vi "Generate LabVIEW FPGA Code for Multistage Multirate Filter.vi"() -> ()   [LabVIEW 2023]
doc: "Demonstrates how to use the DFD FXP NStage MRate Code Generator VI to generate LabVIEW field-programmable gate array (FPGA) code from a fixed-point multistage multirate filter.\n\nComplete the following steps to use this VI.\n1) Specify the <B>Modeling Settings</B>.\n2) Specify a <B>Destination Folder</B> for code generation.\n3) Specify a <B>Filter Name</B> for code generation.\n4) Specify <B># Channels</B> that you want the filter to process.\n5) Specify <B>Open Project?</B> to decide whether to open the generated LabVIEW project or not after code generation.\n6) Run the VI.\n7) Observe the Maximum Input Fs@40 MHz FPGA Clock to obtain information about the processing power of the generated fixed-point multirate filter block."
uses:
  <vilib>/addons/Digital Filter Design/_Objects.llb/DFD Multirate Filtering Mode.ctl
  <vilib>/addons/Digital Filter Design/_Objects.llb/DFD Filter Ripple Specification (Design).ctl
  <vilib>/addons/Digital Filter Design/_Objects.llb/DFD Multirate Filter Specification (Design).ctl
  <vilib>/addons/Digital Filter Design/NI_DigFilterLicensed.lvlib
panel:
  out "Maximum Input Fs@40 MHz FPGA Clock":dbl format="%#_5p Hz"
  out "lvproj Path":path
  in  "Open Project?":bool=TRUE
  in  "Filter Name":string
  in  "# Channels":i32=1
  in  "Destination Folder":path
  out "Error Message":string
  in  "Interstage Word Lengths":i16[](array[numeric])=[16]
  in  "Output Word Length":i16=16
  in  "Input Word Length":i16=16
  # "Select Help>>Show Context Help and move the cursor over the VI icon for more information."
  # "Modeling Settings"
  # "Code Generation Settings"
  # "Code Generation Feedback"
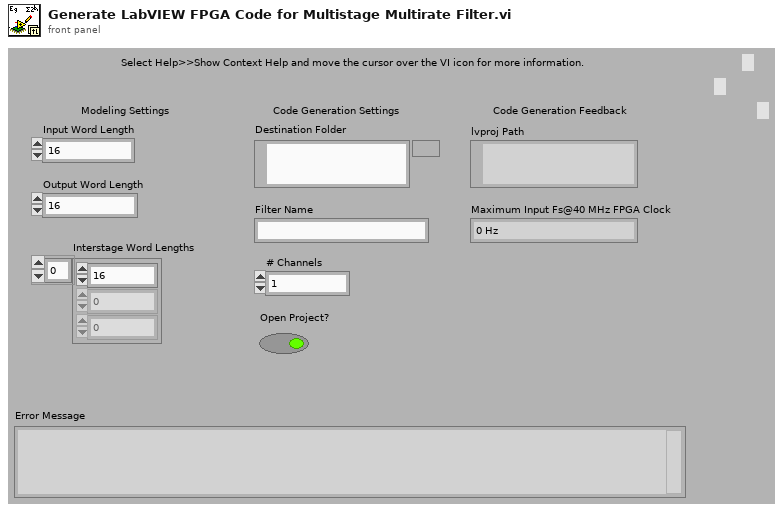
[diagram p1: front panel]
types:
  T1 = typedef "NI_DigFilterLicensed.lvlib/DFD Multirate Filter Specification (Design).ctl" = cluster{"fpass":dbl, "fstop":dbl}
  T2 = typedef "NI_DigFilterLicensed.lvlib/DFD Filter Ripple Specification (Design).ctl" = cluster{"passband":dbl, "stopband":dbl, "dB/linear? (T: dB)":bool}
  T3 = typedef "NI_DigFilterLicensed.lvlib/DFD Multirate Filtering Mode.ctl" = u16
  T4 = typedef "NI_DigFilterLicensed.lvlib/DFD Multirate Filter Obj.ctl" = cluster{"mMRate_Structure":enum16{"CIC", "FIR", "IIR", "Lattice"}, "mMRate_Mode":T5, "mMRate_Factor":i32, "mMRate_FIRParams":cluster{"mMRate_FIR_H":dbl[], "mMRate_FIR_IsNyquist?":bool, "mMRate_FIR_IsSymmetric?":bool}, "mMRate_CICParams":cluster{"mMRate_CIC_#Stage":i32, "mMRate_CIC_Lag":i32, "mMRate_CIC_Type":enum16{"Lowpass", "Highpass"}}, "mMRate_Order":i32, "mMRate_Version":string, "mMRate_Comments":string, "mMRate_RationalFactor":cluster{"mMRate_L":i32, "mMRate_M":i32}, "mMRate_Fs":dbl, "mMRate_Quantized?":bool, "mMRate_QFilterGain":dbl, "mMRate_CoefWl":i16, "mMRate_Scaling":cluster{"mMRate_ScaleByPowerOf2?":bool, "mMRate_ScaleType":T6}, "mMRate_InputWl":i16, "mMRate_OutputWl":i16, "mMRate_OutputMode":T7, "mMRate_MultMode":T8, "mMRate_BitPruning":bool, "mMRate_GainWl":i16, "mMRate_OutputFwl":i16, "mMRate_SumIwl":i16, "mMRate_InputIwl ":i16, "mMRate_SumWl":i16, "mMRate_CoefIwl":i16}
  T5 = typedef "NI_DigFilterLicensed.lvlib/DFD Multirate Mode.ctl" = i16
  T6 = typedef "NI_DigFilterLicensed.lvlib/DFD Coef Norm Type.ctl" = enum16{"No Norm", "Time Domain 1-Norm", "Time Domain 2-Norm", "Time Domain Inf-Norm"}
  T7 = typedef "NI_DigFilterLicensed.lvlib/DFD Round-off Mode.ctl" = enum16{"Nearest", "Truncation"}
  T8 = typedef "NI_DigFilterLicensed.lvlib/DFD FXP MRate Multiply Mode.ctl" = enum16{"Truncated", "Full"}
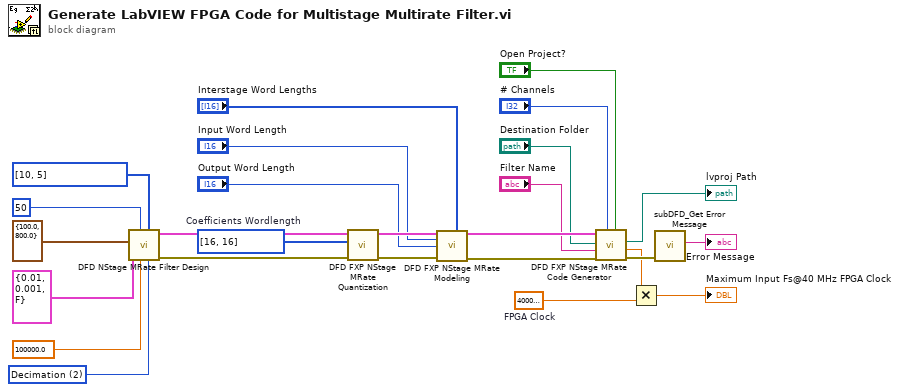
[diagram p0: block diagram]
diagram:
  w4 = 40000000.0  # FPGA Clock
  w18 = i16[] [16, 16]  # Coefficients Wordlength
  w20 = T3 2 items=["No Rate Change", "Interpolation", "Decimation"] ("Filtering Mode")
  n1 = call <vilib>:"DFD NStage MRate Filter Design.vi"("filtering mode"=w20, "manual factorization"=i32[] [10, 5] ("Manual Factorization"), "fs in [Hz]"=100000.0 ("Sampling Rate [Hz]"), "factor"=50 ("Factor"), "ripple specs"=T2 {"passband"=0.01, "stopband"=0.001, "dB/linear? (T: dB)"=FALSE} ("Ripple Specs"), "freq specs [Hz]"=T1 {"fpass"=100.0, "fstop"=800.0} ("Freq Spec")) -> ("error out"=w19:errorcluster, "multirate filters out"=w24:T4[])  [unwired: 2 in, 2 out]
  n2 = call <vilib>:"DFD FXP NStage MRate Quantization.vi"("error in (no error)"=w19, "coefficients word lengths"=w18, "multirate filters in"=w24) -> ("error out"=w3:errorcluster, "multirate filters out"=w17:T4[])  [unwired: 3 in, 4 out]
  n3 = call <vilib>:"DFD FXP NStage MRate Modeling.vi"("interstage word lengths"="Interstage Word Lengths", "error in (no error)"=w3, "output word length"="Output Word Length", "input word length"="Input Word Length", "multirate filters in"=w17) -> ("error out"=w2:errorcluster, "multirate filters out"=w14:T4[])  [unwired: 3 in, 2 out]
  n4 = call <vilib>:"DFD FXP NStage MRate Code Generator.vi"("open project? (F)"="Open Project?", "# channels"="# Channels", "error in (no error)"=w2, "filter name"="Filter Name", "destination folder"="Destination Folder", "multirate filters"=w14) -> ("error out"=w12:errorcluster, "sampling frequency/FPGA clock"=w6:dbl, "lvproj path"=→"lvproj Path":path)  [unwired: 1 in, 2 out]
  n5 = Multiply(x=w6, y=w4) -> (x*y=→"Maximum Input Fs@40 MHz FPGA Clock":dbl)
  n6 = call <vilib>:"subDFD_Get Error Message.vi"("error in (no error)"=w12) -> ("Error Message"=→"Error Message":string)  [unwired: 10 out]
